vi "MHL Cases.vi"(8 "error in":errorcluster, 11 "BaseView in":refnum<class "BaseView.lvclass">) -> (0 "error out":errorcluster, 3 "BaseView out":refnum<class "BaseView.lvclass">)   [LabVIEW 2020, in "BaseView.lvclass"]
doc: "The base class Message Handling Loop cases of a Worker's QMH."
uses:
  BaseView.lvclass
  C:/Program Files (x86)/National Instruments/LabVIEW 2020/vi.lib/addons/_Workers/Library/Classes/Worker/Worker.lvclass
  <vilib>/addons/_Workers/Library/Classes/Worker/Worker.lvclass/Worker.ctl
  <vilib>/addons/_Workers/Library/Classes/Message/Message.lvclass/Message.ctl
  Initialization Data.ctl
  Response Cases.ctl
  BaseView.lvclass/BaseView.ctl
  rqp_InsertPanel.ctl
  <vilib>/addons/_Workers/Library/Classes/Worker/Worker.lvclass
  <vilib>/addons/_Workers/Library/Classes/Message/Message.lvclass
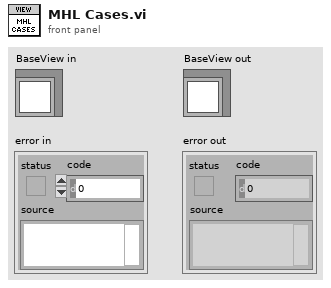
[diagram p1: front panel]
types:
  T1 = typedef "Workers.lvlib/Case Label.ctl" = string
  T2 = typedef "BaseView.lvclass/Initialization Data.ctl" = cluster{"Response Cases":T3}
  T3 = typedef "BaseView.lvclass/Response Cases.ctl" = cluster{"Placeholder - Can be deleted":string}
  T4 = typedef "BaseView.lvclass/rqp_InsertPanel.ctl" = cluster{"SubPanel":refnum<vi>}
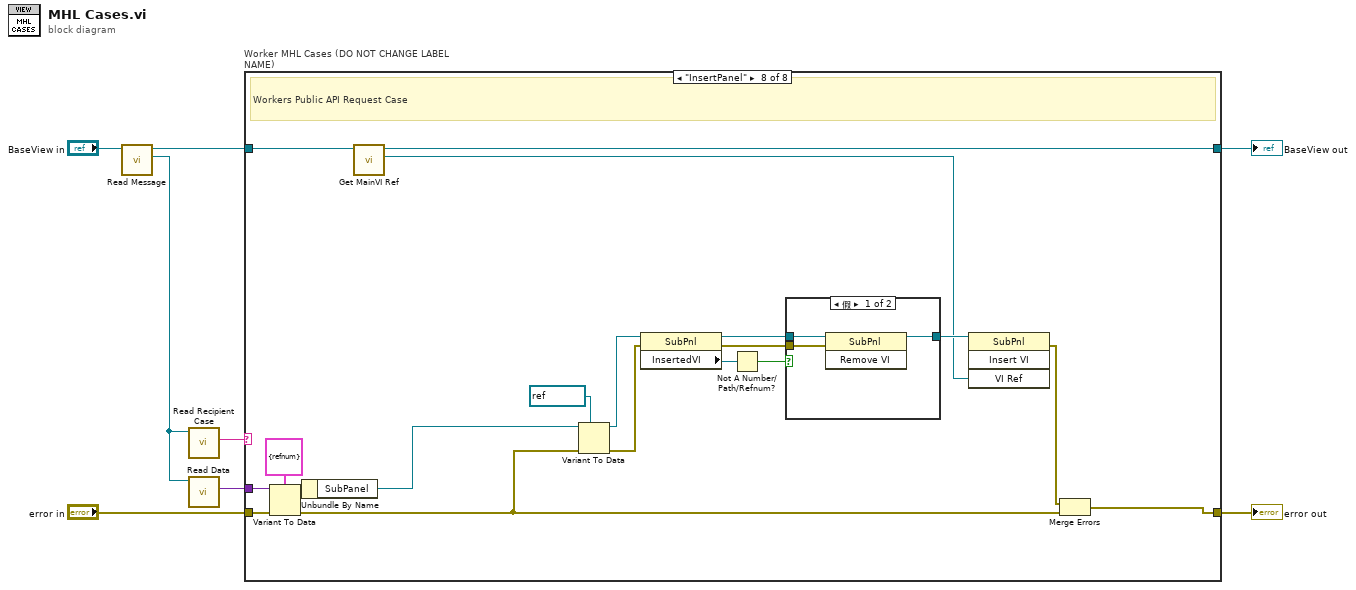
[diagram p0: block diagram]
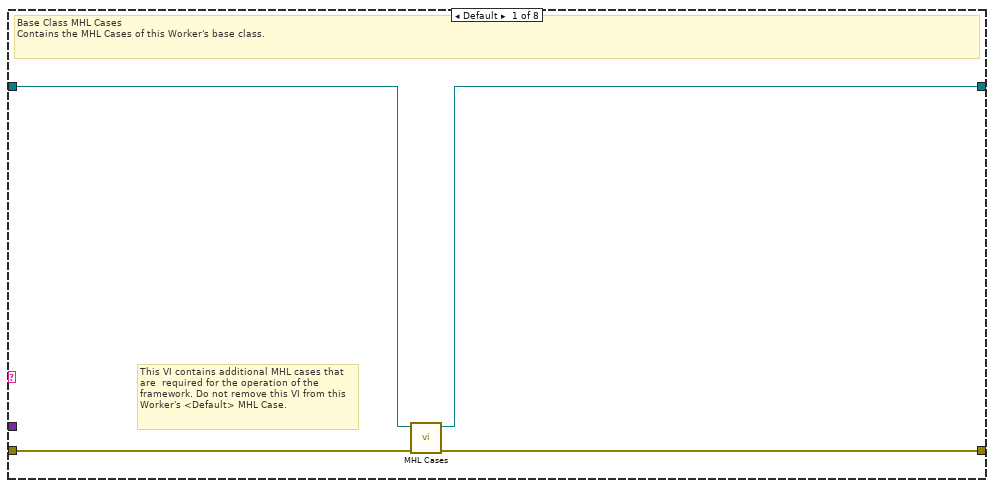
[diagram p2: hidden frame]
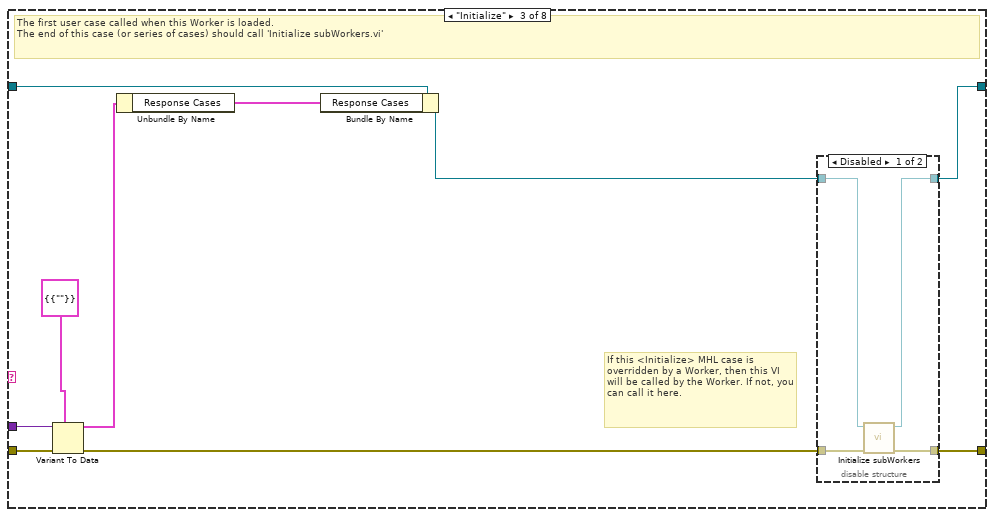
[diagram p4: hidden frame]
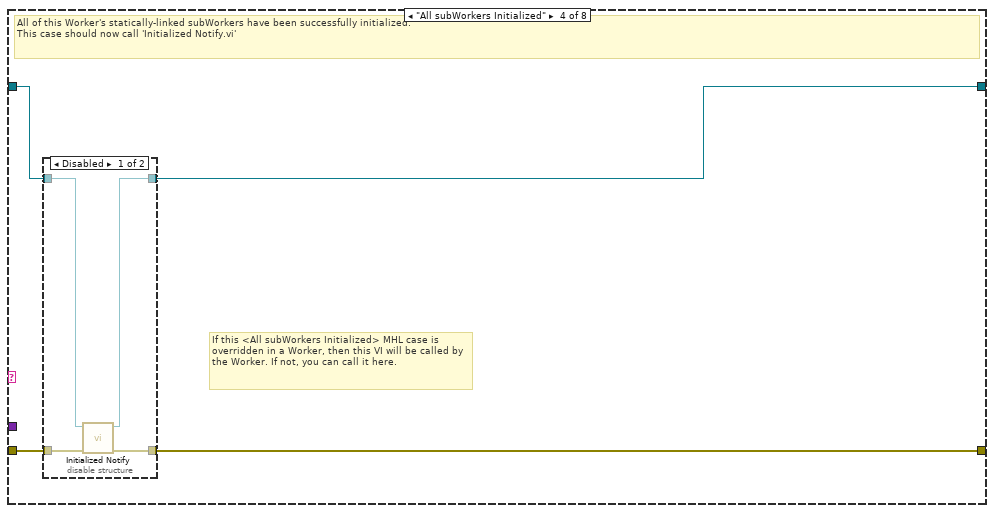
[diagram p6: hidden frame]
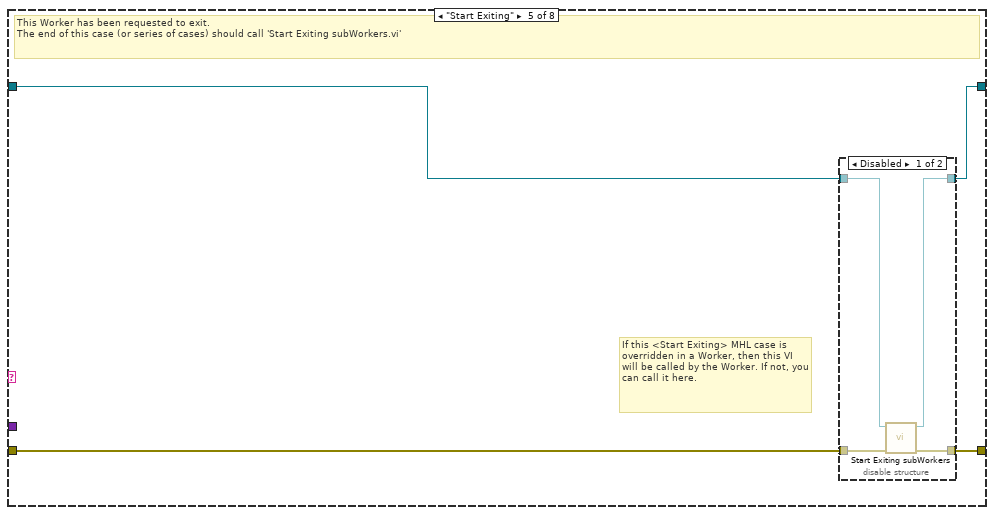
[diagram p8: hidden frame]
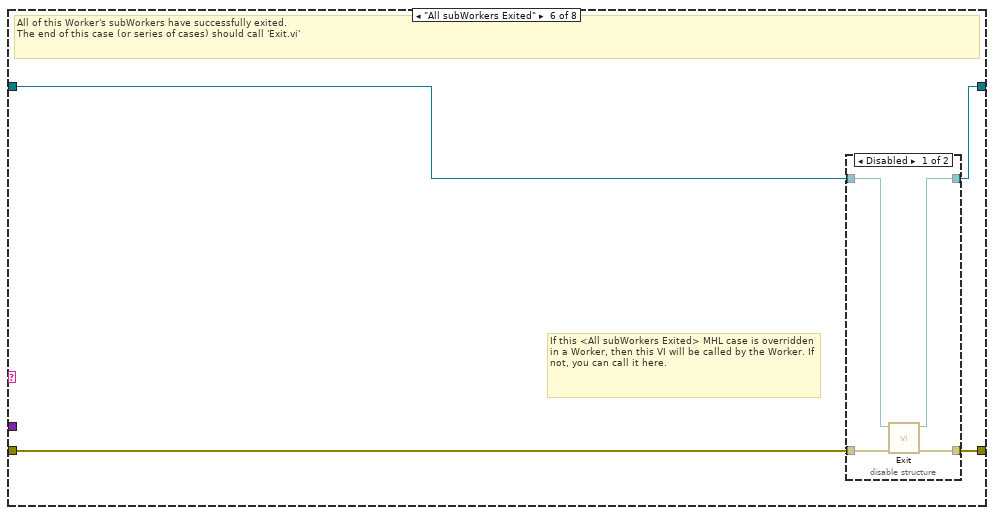
[diagram p10: hidden frame]
diagram:
  n1 = call <vilib>:"Read Message.vi"("Worker"="BaseView in") -> ("Message"=w2:refnum<class "Message.lvclass">, "dup Worker out"=w8:refnum<class "BaseView.lvclass">)  [unwired: 9 in]
  n2 = call <vilib>:"Read Recipient Case.vi"("Message"=w2) -> ("Recipient Case"=w7:T1)  [unwired: 9 in, 1 out]
  n3 = call <vilib>:"Read Data.vi"("Message"=w2) -> ("Data"=w1:variant)  [unwired: 9 in, 1 out]
  n4 = case "Worker MHL Cases (DO NOT CHANGE LABEL NAME)" shown="\"InsertPanel\"" w7 {
    tunnel: [w12 w14 w17 w31 w42 w53 w62 w66] -> w6
    tunnel: [w11 w13 w15 w33 w43 w51 w61 w77] -> w5
    tunnel: "error in" -> [w10 w14 w24 w32 w41 w54 w62 w81]
    tunnel: w8 -> [w9 w13 w23 w34 w44 w52 w61 w76]
    tunnel: w1 -> [_ _ w22 _ _ _ _ w79]
    frame Default {
      # "This VI contains additional MHL cases that are  required for the operation of the framework. Do not remove this VI from this Worker's <Default> MHL Case."
      # "Base Class MHL Cases\nContains the MHL Cases of this Worker's base class."
      n5 = call-parent "MHL Cases.vi"("error in"=w10, "Worker in"=w9) -> ("error out"=w12:errorcluster, "Worker out"=w11:refnum<class "BaseView.lvclass">)  [unwired: 8 in]
    }
    frame "------------ FRAMEWORK CASES -----------" {
      # "Start of Workers Framework Cases"
    }
    frame "Initialize" {
      # "If this <Initialize> MHL case is overridden by a Worker, then this VI will be called by the Worker. If not, you can call it here."
      # "The first user case called when this Worker is loaded.\nThe end of this case (or series of cases) should call 'Initialize subWorkers.vi'"
      n6 = Variant To Data(error in=w24, type=T2 {"Response Cases"={"Placeholder - Can be deleted"=""}} ("Initialization Data"), Variant=w22) -> (data=w21:T2, error out=w18:errorcluster)
      n7 = Unbundle By Name(w21) -> ("Response Cases"=w20:T3)
      n8 = Bundle By Name(cluster=w23, "Response Cases"=w20) -> (w16:refnum<class "BaseView.lvclass">)
      n9 = disable-structure shown="Disabled" {
        disable-tunnel: w18 -> [w28 w29]
        disable-tunnel: [w27 w29] -> w17
        disable-tunnel: w16 -> [w26 w30]
        disable-tunnel: [w25 w30] -> w15
        frame Disabled {
          n10 = call-dynamic "Initialize subWorkers.vi"("error in"=w28, "Worker"=w26) -> ("error out"=w27:errorcluster, "dup Worker out"=w25:refnum<class "BaseView.lvclass">)  [unwired: 8 in]
        }
        frame Enabled {
        }
      }
    }
    frame "All subWorkers Initialized" {
      # "If this <All subWorkers Initialized> MHL case is overridden in a Worker, then this VI will be called by the Worker. If not, you can call it here."
      # "All of this Worker's statically-linked subWorkers have been successfully initialized.\nThis case should now call 'Initialized Notify.vi'"
      n11 = disable-structure shown="Disabled" {
        disable-tunnel: w34 -> [w38 w40]
        disable-tunnel: [w37 w40] -> w33
        disable-tunnel: w32 -> [w36 w39]
        disable-tunnel: [w35 w39] -> w31
        frame Disabled {
          n12 = call-dynamic "Initialized Notify.vi"("error in"=w36, "Worker"=w38) -> ("error out"=w35:errorcluster, "dup Worker out"=w37:refnum<class "BaseView.lvclass">)  [unwired: 8 in]
        }
        frame Enabled {
        }
      }
    }
    frame "Start Exiting" {
      # "If this <Start Exiting> MHL case is overridden in a Worker, then this VI will be called by the Worker. If not, you can call it here."
      # "This Worker has been requested to exit. \nThe end of this case (or series of cases) should call 'Start Exiting subWorkers.vi'"
      n13 = disable-structure shown="Disabled" {
        disable-tunnel: w44 -> [w48 w50]
        disable-tunnel: [w47 w50] -> w43
        disable-tunnel: [w46 w49] -> w42
        disable-tunnel: w41 -> [w45 w49]
        frame Disabled {
          n14 = call-dynamic "Start Exiting subWorkers.vi"("error_in"=w45, "Worker"=w48) -> ("error out"=w46:errorcluster, "dup Worker out"=w47:refnum<class "BaseView.lvclass">)  [unwired: 8 in]
        }
        frame Enabled {
        }
      }
    }
    frame "All subWorkers Exited" {
      # "If this <All subWorkers Exited> MHL case is overridden in a Worker, then this VI will be called by the Worker. If not, you can call it here."
      # "All of this Worker's subWorkers have successfully exited. \nThe end of this case (or series of cases) should call 'Exit.vi'"
      n15 = disable-structure shown="Disabled" {
        disable-tunnel: w54 -> [w58 w59]
        disable-tunnel: [w57 w59] -> w53
        disable-tunnel: w52 -> [w56 w60]
        disable-tunnel: [w55 w60] -> w51
        frame Disabled {
          n16 = call-dynamic "Exit.vi"("error_in"=w58, "Worker"=w56) -> ("error out"=w57:errorcluster, "dup Worker out"=w55:refnum<class "BaseView.lvclass">)  [unwired: 8 in]
        }
        frame Enabled {
        }
      }
    }
    frame "------------- PUBLIC API CASES -------------" {
      # "Start of Workers Public API Cases"
    }
    frame "InsertPanel" {
      # "Workers Public API Request Case"
      n17 = Variant To Data(error in=w81, type=T4 {"SubPanel"=refnum} ("Data"), Variant=w79) -> (data=w78:T4, error out=w64:errorcluster)
      n18 = Unbundle By Name(w78) -> ("SubPanel"=w65:refnum<vi>)
      n19 = call-dynamic "Get MainVI Ref.vi"("Worker_"=w76) -> ("MainVI Ref"=w63:refnum<vi>, "dup Worker_out"=w77:refnum<class "BaseView.lvclass">)  [unwired: 8 in, 1 out]
      n20 = Variant To Data(error in=w64, type=refnum<vi> refnum ("子面板"), Variant=w65) -> (data=w74:refnum<vi>, error out=w67:errorcluster)
      n21 = property class="SubPnl"(reference=w74, error in=w67) -> (reference out=w71:refnum<vi>, error out=w72:errorcluster, "InsertedVI"=w70:refnum<vi>)
      n22 = Not A Number/Path/Refnum?(number/path/refnum=w70) -> (NaN/Path/Refnum?=w73:bool)
      n23 = case shown="假" w73 {
        tunnel: w71 -> [w84 w85]
        tunnel: w72 -> [w83 _]
        tunnel: [w82 w85] -> w75
        frame False {
          n24 = invoke class="SubPnl" method="Remove VI"(reference=w84, error in=w83) -> (reference out=w82:refnum<vi>)  [unwired: 1 in, 2 out]
        }
        frame True {
        }
      }
      n25 = invoke class="SubPnl" method="Insert VI"(reference=w75, "VI Ref"=w63) -> (error out=w68:errorcluster)  [unwired: 2 in, 3 out]
      n26 = Merge Errors(w68, w64) -> (w66:errorcluster)
    }
  }
  "BaseView out" <- w5
  "error out" <- w6
